vi "x-axis.vi"(8 "error in (no error)":errorcluster, 11 "Translation Stage in":refnum<class "Translation Stage.lvclass">) -> (0 "error out":errorcluster, 1 "Label":string, 2 "Unit":string, 3 "Translation Stage out":refnum<class "Translation Stage.lvclass">)   [LabVIEW 2015, in "Translation Stage.lvclass"]
uses:
  Translation Stage.lvclass
  Scanner/Scanner.lvclass
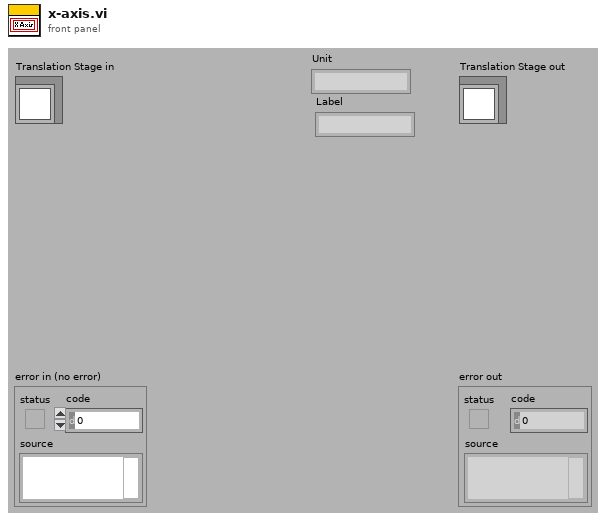
[diagram p1: front panel]
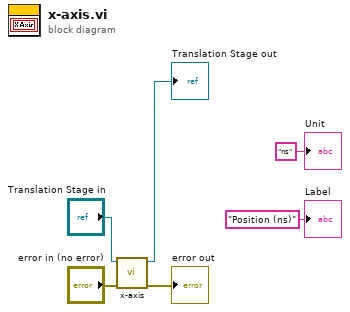
[diagram p0: block diagram]
diagram:
  n1 = call-parent "x-axis.vi"("error in (no error)"="error in (no error)", "Scanner in"="Translation Stage in") -> ("error out"=→"error out":errorcluster, "Scanner out"=→"Translation Stage out":refnum<class "Translation Stage.lvclass">)  [unwired: 6 in, 2 out]
  "Label" <- "Position (ns)" ("Label")
  "Unit" <- "ns" ("Unit")
